vi "AFG3352X.initialize.vi"(0 "i ref in":refnum<vi>, 1 "queryID":bool, 2 "resetDevice":bool, 3 "ms timeout (10000)":i32=10000, 5 "error in (no error)":errorcluster) -> (14 "i ref out":refnum<vi>, 16 "deviceID":string, 17 "timed out":bool, 19 "error out":errorcluster)   [LabVIEW 2014, in "AFG3352X.lvlib"]
doc: "(Re)initializs the device."
uses:
  AFG3352X.lvlib
  CSCore/CSApplicationBaseClasses/DeviceBase/DeviceBase.lvlib
  CSinstr.lib/Agilent 3352X Series/Agilent 3352X Series.lvlib
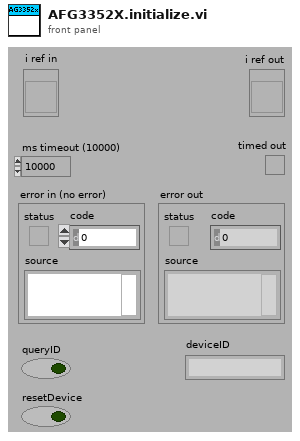
[diagram p1: front panel]
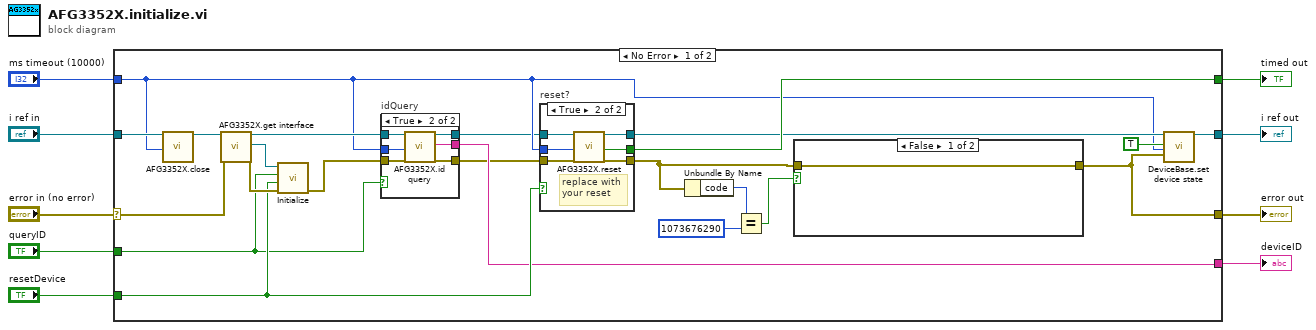
[diagram p0: block diagram]
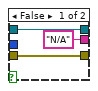
[diagram p3: hidden frame]
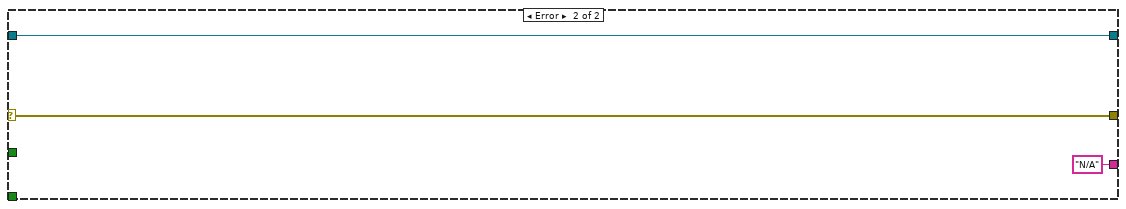
[diagram p5: hidden frame]
diagram:
  n1 = case shown="No Error" "error in (no error)" {
    selector: "error in (no error)" -> [w25 w51]
    tunnel: [w31 _] -> w9
    tunnel: [w28 w52] -> w8
    tunnel: "ms timeout (10000)" -> [w19 _]
    tunnel: "i ref in" -> [w30 w52]
    tunnel: "queryID" -> [w18 _]
    tunnel: [w10 w51] -> w3
    tunnel: "resetDevice" -> [w22 _]
    tunnel: [w17 "N/A"] -> w1
    frame No Error {
      n2 = call "AFG3352X.close.vi"("i ref in"=w30, "ms timeout (10000)"=w19) -> ("i ref out"=w26:refnum<vi>)  [unwired: 15 in, 2 out]
      n3 = call "AFG3352X.get interface.vi"("i ref in"=w26, "error in (no error)"=w25) -> ("i ref out"=w21:refnum<vi>, "interface"=w24:refnum<visa-resource-name>, "error out"=w23:errorcluster)  [unwired: 15 in]
      n4 = call "Initialize.vi"("error in (no error)"=w23, "Reset (Enable)"=w22, "ID Query (Enable)"=w18, "VISA resource name"=w24) -> ("error out"=w20:errorcluster)  [unwired: 6 in, 1 out]
      n5 = case "idQuery" shown="True" w18 {
        tunnel: w21 -> [w35 w41]
        tunnel: w20 -> [w34 w40]
        tunnel: w19 -> [_ w39]
        tunnel: [w35 w38] -> w16
        tunnel: [w34 w37] -> w15
        tunnel: ["N/A" ("IDString") w36] -> w17
        frame False {
        }
        frame True {
          n6 = call "AFG3352X.id query.vi"("i ref in"=w41, "ms timeout (10000)"=w39, "error in (no error)"=w40) -> ("i ref out"=w38:refnum<vi>, "IDString"=w36:string, "error out"=w37:errorcluster)  [unwired: 13 in, 1 out]
        }
      }
      n7 = case "reset?" shown="True" w22 {
        tunnel: w16 -> [w43 w49]
        tunnel: w15 -> [w42 w48]
        tunnel: w19 -> [_ w47]
        tunnel: [_ w46] -> w31
        tunnel: [w42 w45] -> w11
        tunnel: [w43 w44] -> w29
        frame False {
        }
        frame True {
          # "replace with\nyour reset"
          n8 = call "AFG3352X.reset.vi"("i ref in"=w49, "ms timeout (10000)"=w47, "error in (no error)"=w48) -> ("i ref out"=w44:refnum<vi>, "timed out"=w46:bool, "error out"=w45:errorcluster)  [unwired: 14 in]
        }
      }
      n9 = Unbundle By Name(w11) -> ("code"=w14:i32)
      n10 = Equal?(x=w14, y=1073676290) -> (x = y?=w12:bool)
      n11 = case shown="False" w12 {
        tunnel: w11 -> [w32 _]
        tunnel: [w32 _] -> w10
        frame False {
        }
        frame True {
        }
      }
      n12 = call "DeviceBase.set device state.vi"("i ref in"=w29, "implicit"=TRUE, "ms timeout (10000)"=w19, "device error"=w10) -> ("i ref out"=w28:refnum<vi>)  [unwired: 13 in, 2 out]
    }
    frame Error {
    }
  }
  "error out" <- w3
  "i ref out" <- w8
  "timed out" <- w9
  "deviceID" <- w1
